vi "OscTestPic.vi"() -> ()   [LabVIEW 2017]
uses:
  <vilib>/Analysis/baseanly.llb/Mean (DBL).vi
  DS1054z.lvlib
  <vilib>/Analysis/NI_AALBase.lvlib
panel:
  out "Waveform Chart":u32(graph)
  out "Array":string[](array[string])
  out "OutData":cluster{string, "userdata":string}
  out "Waveform Graph 4":u32[](graph)
  out "mean":dbl format="%0.2f"
  out "Waveform Graph 3":dbl[](graph)
  out "Numeric":i32
  out "x-y":u32
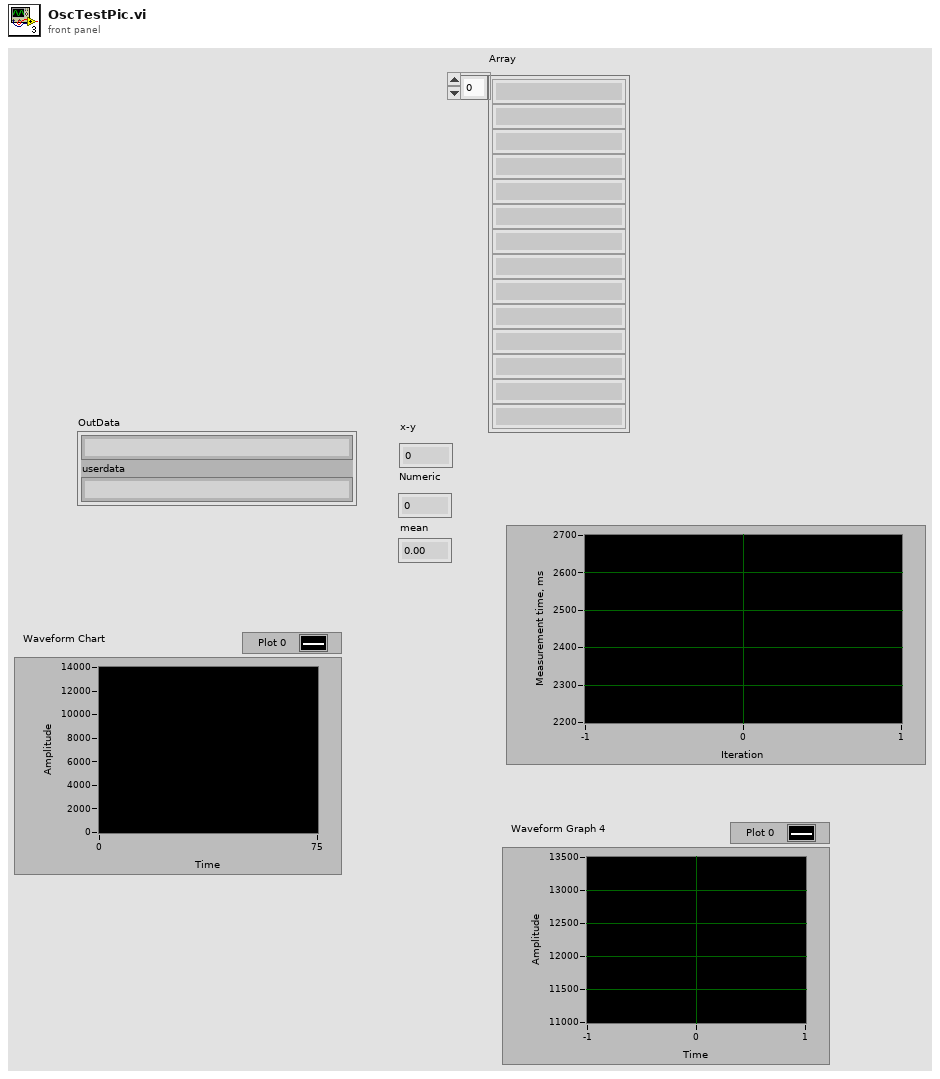
[diagram p1: front panel]
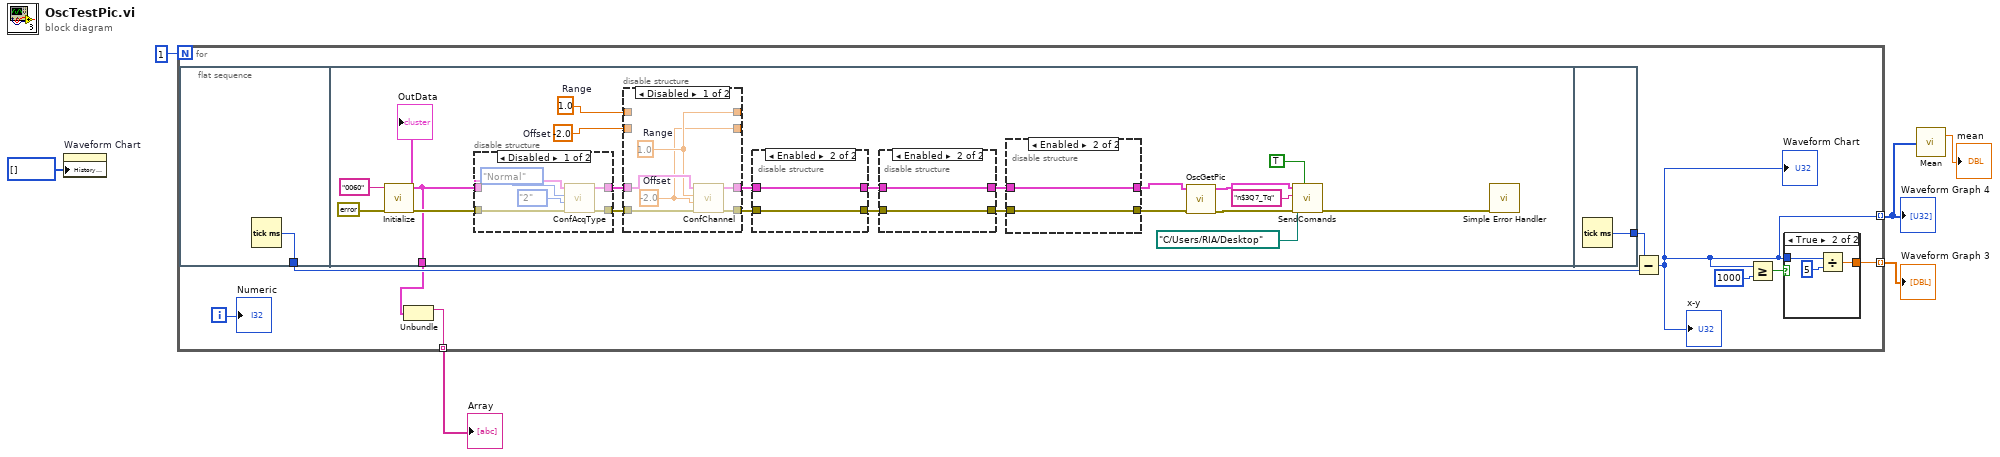
[diagram p0: block diagram]
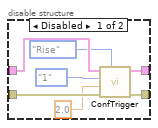
[diagram p3: hidden frame]
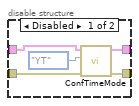
[diagram p4: hidden frame]
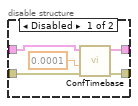
[diagram p5: hidden frame]
diagram:
  n1 = property on="Waveform Chart" class="WFChart (strict)"("History Data"=u32[] []) -> ()  [unwired: 2 in, 2 out]
  n2 = for {
    N: 1 -> [_]
    tunnel: [w7] -> w1 mode=indexing
    tunnel: [w11] -> w4 mode=indexing
    tunnel: [w9] -> w3 mode=indexing
    i -> [w14]
    n3 = flat-sequence {
      tunnel: [w20] -> w15
      tunnel: [w28] -> w10
      tunnel: [w84] -> w8
      frame #0 {
        n4 = Tick Count (ms)() -> (millisecond timer value=w20:u32)
      }
      frame #1 {
        w29 = -2.0  # Offset
        w30 = 1.0  # Range
        n5 = call "Initialize.vi"("error in (no error)"=errorcluster {"status"=FALSE, "code"=0, "source"=""}, "UserID"="0060") -> ("error out"=w40:errorcluster, "OutData"=w28:cluster{string, "userdata":string})  [unwired: 8 in]
        "OutData" <- w28
        n6 = disable-structure shown="Disabled" {
          disable-tunnel: w28 -> [w81 w83]
          disable-tunnel: w40 -> [w80 w82]
          disable-tunnel: [w77 w83] -> w38
          disable-tunnel: [w76 w82] -> w37
          frame Disabled {
            n7 = call "ConfAcqType.vi"("error in"=w80, "NumOfAver"=enum16{"2", "4", "8", "16"}."2", "Type"=enum16{"Normal", "Average", "Peak Detect"}."Normal", "InputData"=w81) -> ("error out"=w76:errorcluster, "OutputData"=w77:cluster{"String":string, string})  [unwired: 6 in]
          }
          frame Enabled {
          }
        }
        n8 = disable-structure shown="Disabled" {
          disable-tunnel: w38 -> [w71 w75]
          disable-tunnel: w37 -> [w70 w74]
          disable-tunnel: [w69 w75] -> w36
          disable-tunnel: [w68 w74] -> w35
          disable-tunnel: [w67 w73] -> _
          disable-tunnel: [w66 w72] -> _
          disable-tunnel: w30 -> [_ w73]
          disable-tunnel: w29 -> [_ w72]
          frame Disabled {
            w66 = -2.0  # Offset
            w67 = 1.0  # Range
            n9 = call "ConfChannel.vi"("error in"=w70, "Offset"=w66, "Range"=w67, "InputData"=w71) -> ("error out"=w68:errorcluster, "OutputData"=w69:cluster{"String":string, string})  [unwired: 6 in]
          }
          frame Enabled {
          }
        }
        n10 = disable-structure shown="Enabled" {
          disable-tunnel: w36 -> [w63 w65]
          disable-tunnel: w35 -> [w62 w64]
          disable-tunnel: [w61 w65] -> w34
          disable-tunnel: [w60 w64] -> w33
          frame Disabled {
            n11 = call "ConfTimebase.vi"("error in"=w62, "Timebase"=0.0001, "InputData"=w63) -> ("error out"=w60:errorcluster, "OutputData"=w61:cluster{"String":string, string})  [unwired: 7 in]
          }
          frame Enabled {
          }
        }
        n12 = disable-structure shown="Enabled" {
          disable-tunnel: w34 -> [w56 w58]
          disable-tunnel: w33 -> [w55 w57]
          disable-tunnel: [w54 w58] -> w32
          disable-tunnel: [w53 w57] -> w31
          frame Disabled {
            n13 = call "ConfTimeMode.vi"("error in"=w55, "Timebase Mode"=enum16{"YT", "XY"}."YT", "InputData"=w56) -> ("error out"=w53:errorcluster, "OutputData"=w54:cluster{"String":string, string})  [unwired: 7 in]
          }
          frame Enabled {
          }
        }
        n14 = disable-structure shown="Enabled" {
          disable-tunnel: [w49 w51] -> w25
          disable-tunnel: [w48 w50] -> w24
          disable-tunnel: w32 -> [w47 w51]
          disable-tunnel: w31 -> [w46 w50]
          frame Disabled {
            n15 = call "ConfTrigger.vi"("Slope"=enum16{"Rise", "Fall", "Both"}."Rise", "error in"=w46, "Level"=2.0, "Source"=enum16{"1", "2", "3", "4"}."1", "InputData"=w47) -> ("error out"=w48:errorcluster, "OutputData"=w49:cluster{"String":string, string})  [unwired: 5 in]
          }
          frame Enabled {
          }
        }
        n16 = call "OscGetPic.vi"("error in"=w24, "InputData"=w25) -> ("error out"=w26:errorcluster, "OutputData"=w27:cluster{"String":string, string})  [unwired: 8 in]
        n17 = call "SendComands.vi"("GetPicture?"=TRUE, "error in (no error)"=w26, "output file directory"=path "C:/Users/RIA/Desktop", "Password"="n$3Q7_Tq", "InputData"=w27) -> ("error out"=w23:errorcluster)  [unwired: 4 in, 2 out]
        n18 = call <vilib>:"Simple Error Handler.vi"("error in (no error)"=w23) -> ()  [unwired: 4 in, 5 out]
      }
      frame #2 {
        n19 = Tick Count (ms)() -> (millisecond timer value=w84:u32)
      }
    }
    n20 = Unbundle(w10) -> (w9:string)  [unwired: 1 out]
    n21 = Subtract(x=w8, y=w15) -> (x-y=w7:u32)
    "x-y" <- w7
    "Waveform Chart" <- w7
    n22 = Greater Or Equal?(x=w7, y=u32 1000) -> (x >= y?=w12:bool)
    n23 = case shown="True" w12 {
      tunnel: w7 -> [w16 w19]
      tunnel: [w16 w17] -> w11
      frame False {
      }
      frame True {
        n24 = Divide(x=w19, y=u32 5) -> (x/y=w17:dbl)
      }
    }
    "Numeric" <- w14
  }
  "Waveform Graph 3" <- w4
  "Waveform Graph 4" <- w1
  "Array" <- w3
  n25 = call-poly <vilib>:"Mean.vi"("X"=w1) -> ("mean"=→"mean":dbl)  [unwired: 1 out]
